vi "export to report file.vi"() -> ()   [LabVIEW 2018, in "Application.lvlib"]
uses:
  Application.lvlib
panel:
  in  "SAP ID":string="SapID"
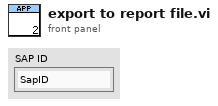
[diagram p1: front panel]
types:
  T1 = enum16{"open", "replace", "create", "open or create", "replace or create", "replace or create with confirmation"}
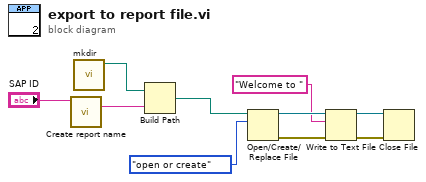
[diagram p0: block diagram]
diagram:
  n1 = call "Create report name.vi"("SAP ID"="SAP ID") -> ("filename"=w8:string)  [unwired: 10 in]
  n2 = call "mkdir.vi"() -> ("created path"=w9:path)  [unwired: 10 in, 1 out]
  n3 = Build Path(base path=w9, name or relative path=w8) -> (appended path=w7:path)
  n4 = Open/Create/Replace File(file path (use dialog)=w7, operation (0:open)=T1."open or create") -> (refnum out=w5:refnum<file>, error out=w4:errorcluster)  [unwired: 4 in, 1 out]
  n5 = Write to Text File(file (use dialog)=w5, text="Welcome to ", error in=w4) -> (refnum out=w2:refnum<file>, error out=w3:errorcluster)  [unwired: 1 in, 1 out]
  n6 = Close File(refnum=w2, error in=w3) -> ()  [unwired: 2 out]
